vi "PicoScope6000ExampleStreaming.vi"() -> ()   [LabVIEW 2016]
uses:
  PS6000.dll
  Wrapper/ps6000Wrap/Release/ps6000Wrap.dll
panel:
  out "Triggered":bool
  in  "Acquisition Settings":T1={"Auto Stop"=TRUE, "Desired Sample Interval"=1, "Pre-trigger Samples"=0, "Post-trigger Samples"=1000000, "Down-Sample Ratio"=1, "Down-Sample Mode"=0, "Overview Buffer Size"=50000, "Time Units"=3} {"Time Units" items=["Nanoseconds (ns)"=2, "Microseconds (us)"=3, "Milliseconds (ms)"=4, "Seconds (s)"=5]; "Down-Sample Mode" items=["None"=0, "Aggregate"=1, "Average"=2, "Decimate"=4, "Distribution"=8]}
  in  "Channel A Settings":T2={"Enabled"=TRUE, "Coupling"=1, "Range"=7, "Analogue Offset"=0.0, "Bandwidth"=0} {"Bandwidth" items=["Full", "20 MHz"]; "Range" items=["10 mV", "20 mV", "50 mV", "100 mV", "200 mV", "500 mV", "1 V", "2 V", "5 V", "10 V", "20 V", "50 V ", "100 V"]; "Coupling" items=["AC", "DC 1 MOhm", "DC 50 Ohm"]}
  out "Sample Interval":u32
  out "Total Samples":u32
  in  "Trigger Settings":T3={"Trigger Enabled"=TRUE, "Trigger Source"=enum."Channel A", "Trigger Threshold (16-bit counts)"=0, "Trigger Direction"=2, "Trigger Delay (samples)"=0, "Auto Trigger Time (ms)"=5000} {"Trigger Direction" items=["Rising"=2, "Falling"=3]}
  out "Auto Stopped":bool
  in  "Apply Settings":bool
  out "Channel A":i16[](graph)
  in  "stop":bool
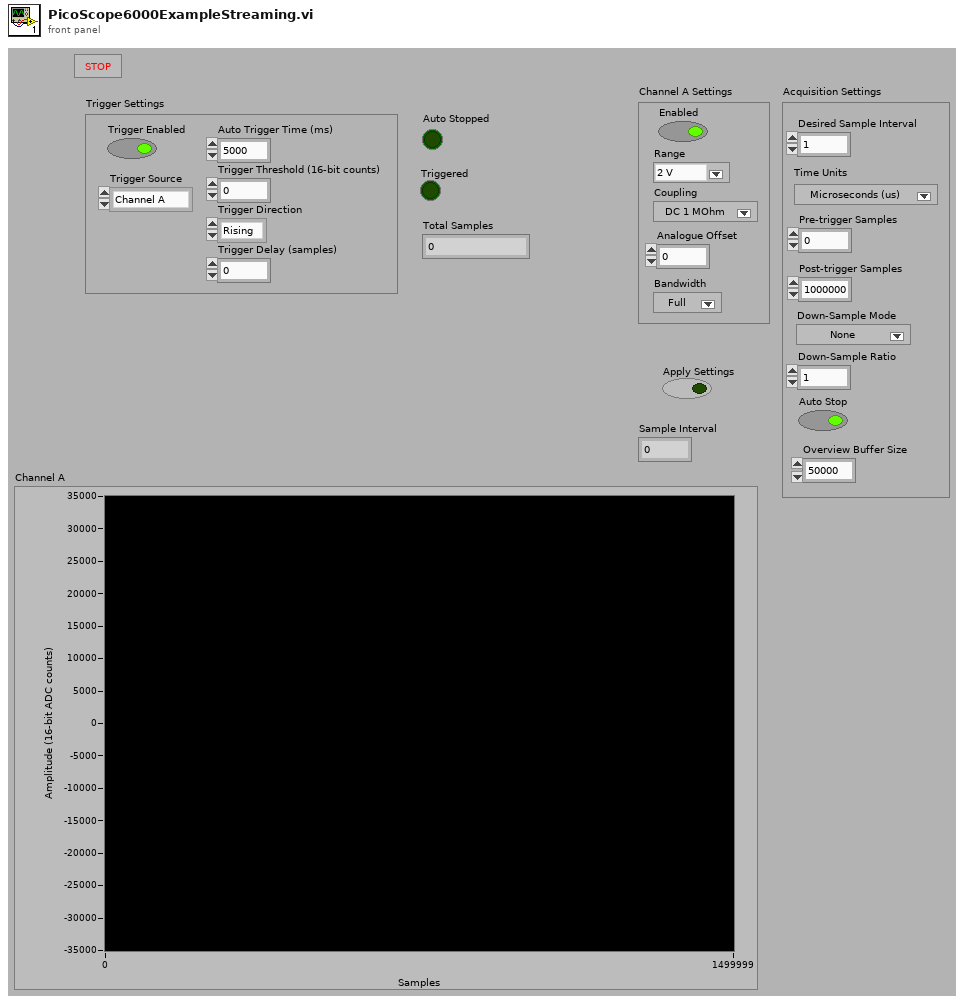
[diagram p1: front panel]
types:
  T1 = cluster{"Auto Stop":bool, "Desired Sample Interval":u32, "Pre-trigger Samples":u32, "Post-trigger Samples":u32, "Down-Sample Ratio":u32, "Down-Sample Mode":u32, "Overview Buffer Size":u32, "Time Units":u32}
  T2 = cluster{"Enabled":bool, "Coupling":u32, "Range":u32, "Analogue Offset":sgl, "Bandwidth":u32}
  T3 = cluster{"Trigger Enabled":bool, "Trigger Source":enum32{"Channel A", "Channel B", "Channel C", "Channel D"}, "Trigger Threshold (16-bit counts)":i16, "Trigger Direction":u16, "Trigger Delay (samples)":u32, "Auto Trigger Time (ms)":i16}
  T4 = cluster{"Enabled":bool, "Coupling":i32, "Range":u16, "Analogue Offset":sgl, "Bandwidth":i32}
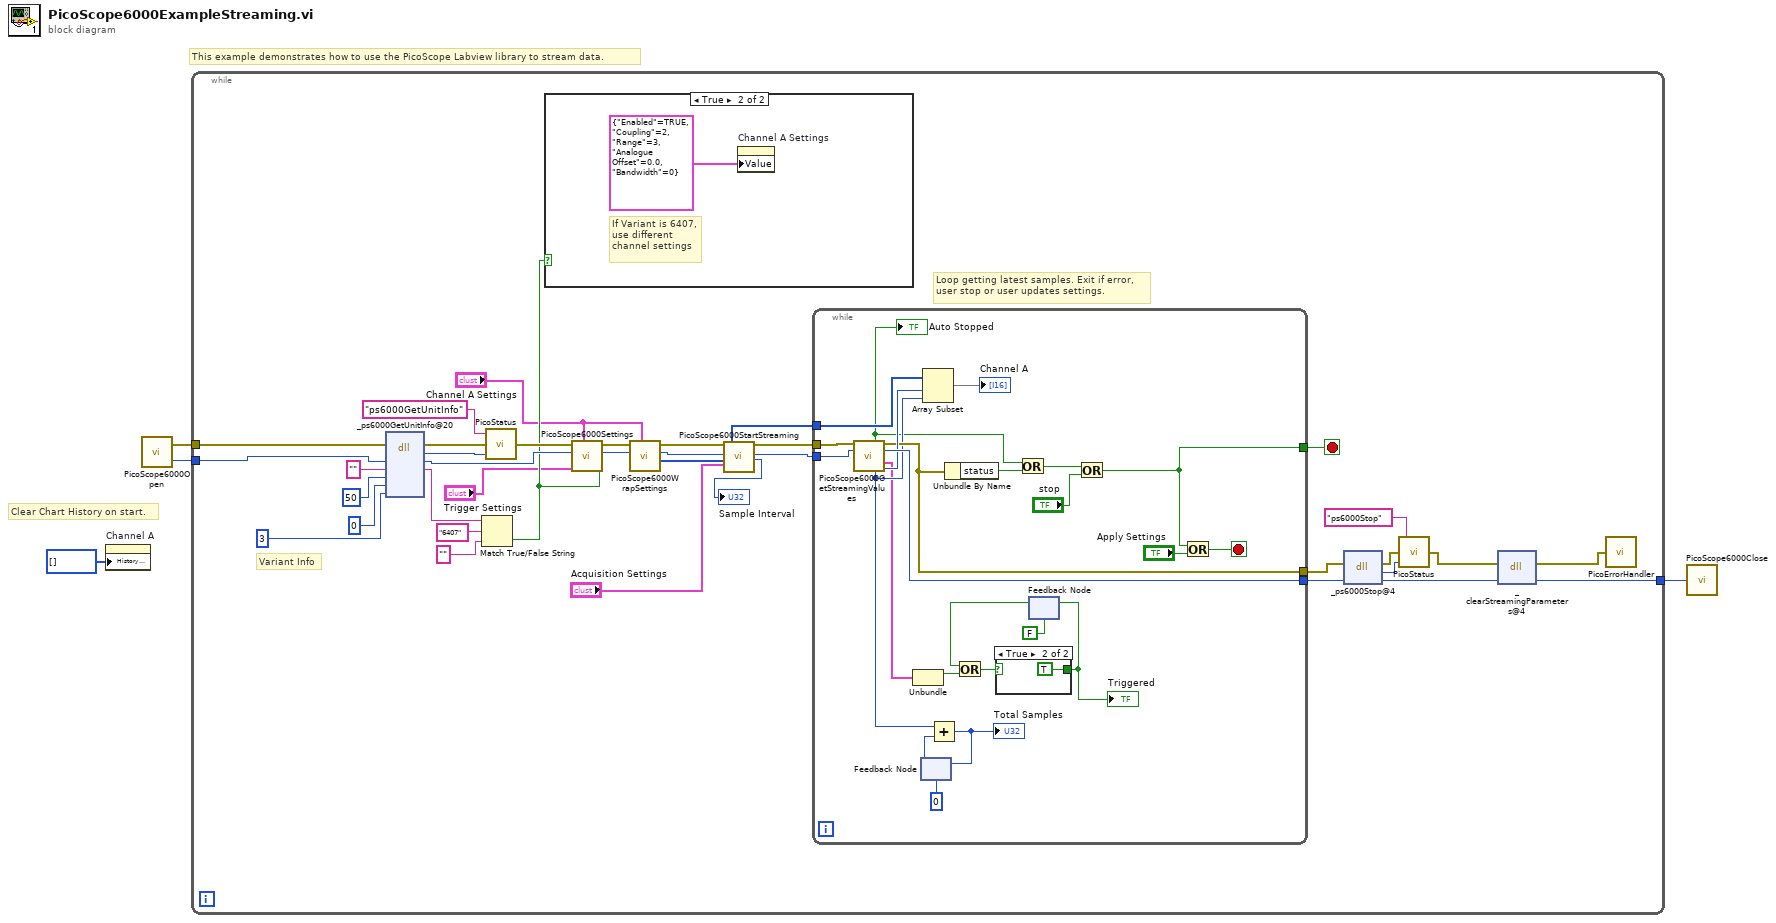
[diagram p0: block diagram]
diagram:
  # "Clear Chart History on start."
  # "This example demonstrates how to use the PicoScope Labview library to stream data."
  n1 = property on="Channel A" class="WFChart (strict)"("History Data"=i16[] []) -> ()  [unwired: 2 in, 2 out]
  n2 = call "PicoScope6000Open.vi"() -> ("error out"=w4:errorcluster, "handle"=w3:i16)  [unwired: 1 in]
  n3 = while {
    tunnel: [w8] -> w2
    tunnel: w4 -> [w27]
    tunnel: w3 -> [w26]
    stop <- w41 stop-if-true
    # "Variant Info"
    # "Loop getting latest samples. Exit if error, \nuser stop or user updates settings."
    n4 = dll-call lib="PS6000.dll" fn="_ps6000GetUnitInfo@20"(error in=w27, "handle"=w26, "string"="", "stringLength"=i16 50, "reqSize"=i16 0, "PICO_INFO"=u32 3 ("info")) -> (error out=w31:errorcluster, "PICO_STATUS"=w30:u32, "handle"=w25:i16, "string"=w28:string)  [unwired: 5 in, 1 out]
    n5 = Match True/False String(2:"" ("false string"), 3:"6407" ("true string"), 4:w28) -> (0:w23:bool)  [unwired: 1 out]
    n6 = call "PicoStatus.vi"("PICO STATUS"=w30, "error in"=w31, "source"="ps6000GetUnitInfo") -> ("error out"=w24:errorcluster)
    n7 = case shown="True" w23 {
      frame False {
      }
      frame True {
        # "If Variant is 6407,\nuse different \nchannel settings"
        n8 = property on="Channel A Settings" class="Clust (strict)"("Value"=T4 {"Enabled"=TRUE, "Coupling"=2, "Range"=3, "Analogue Offset"=0.0, "Bandwidth"=0} ("Channel A Settings")) -> ()  [unwired: 2 in, 2 out]
      }
    }
    n9 = call "PicoScope6000Settings.vi"("PS6407?"=w23, "Channel A Settings"="Channel A Settings", "Trigger Settings"="Trigger Settings", "handle in"=w25, "error in"=w24) -> ("handle out"=w15:i16, "error out"=w17:errorcluster)  [unwired: 5 in]
    n10 = call "PicoScope6000WrapSettings.vi"("Channel A Settings"="Channel A Settings", "Handle In"=w15, "error in (no error)"=w17) -> ("enabledChannels"=w5:i16[], "Handle Out"=w14:i16, "error out"=w16:errorcluster)  [unwired: 6 in]
    n11 = call "PicoScope6000StartStreaming.vi"("error in"=w16, "handle in"=w14, "Enabled Channels"=w5, "Acquisition Settings"="Acquisition Settings") -> ("Channel A"=w38:i16[], "error out"=w40:errorcluster, "handle out"=w39:i16, "Sample Interval"=→"Sample Interval":u32)  [unwired: 5 in, 7 out]
    n12 = while {
      tunnel: w40 -> [w60]
      tunnel: [w59] -> w22
      tunnel: [w64] -> w41
      tunnel: w38 -> [w62]
      tunnel: w39 -> [w61]
      tunnel: [w55] -> w21
      stop <- w63 stop-if-true
      n13 = call "PicoScope6000GetStreamingValues.vi"("error in"=w60, "handle in"=w61) -> ("Auto Stopped"=w50:bool, "error out"=w55:errorcluster, "handle out"=w59:i16, "Trigger"=w44:cluster{bool, "triggeredAt":u32}, "Number of Samples"=w52:u32, "Start Index"=w58:u32)  [unwired: 8 in]
      "Auto Stopped" <- w50
      n14 = Unbundle(w44) -> (w45:bool)  [unwired: 1 out]
      n15 = feedback #1(u32 0) -> (w53:u32)
      n16 = Array Subset(array=w62, index=w58, length=w52) -> (→"Channel A":i16[])
      n17 = Add(x=w52, y=w53) -> (x+y=w51:u32)
      "Total Samples" <- w51
      n18 = feedback-in #1(w51) -> ()
      n19 = Unbundle By Name(w55) -> ("status"=w56:bool)
      n20 = Or(x=w50, y=w56) -> (x .or. y?=w57:bool)
      n21 = feedback #2(FALSE) -> (w48:bool)
      n22 = Or(x=w48, y=w45) -> (x .or. y?=w47:bool)
      n23 = case shown="True" w47 {
        selector: w47 -> [w67 _]
        tunnel: [w67 TRUE] -> w49
        frame False {
        }
        frame True {
        }
      }
      "Triggered" <- w49
      n24 = feedback-in #2(w49) -> ()
      n25 = Or(x=w57, y="stop") -> (x .or. y?=w64:bool)
      n26 = Or(x=w64, y="Apply Settings") -> (x .or. y?=w63:bool)
    }
    n27 = dll-call lib="PS6000.dll" fn="_ps6000Stop@4"(error in=w21, "handle"=w22) -> (error out=w20:errorcluster, "PICO_STATUS"=w19:u32, "handle"=w9:i16)  [unwired: 2 in, 1 out]
    n28 = call "PicoStatus.vi"("PICO STATUS"=w19, "error in"=w20, "source"="ps6000Stop") -> ("error out"=w11:errorcluster)
    n29 = dll-call lib="D:/SoftwareFiles/LabVIEW Files/Picoscope/picoscope-master/sdk/6000/Wrapper/ps6000Wrap/Release/ps6000Wrap.dll" fn="_clearStreamingParameters@4" label="clearStreamingParameters"(error in=w11, "handle"=w9) -> (error out=w10:errorcluster, "handle"=w8:i16)  [unwired: 3 in, 1 out]
    n30 = call "PicoErrorHandler.vi"("error in"=w10) -> ()  [unwired: 1 out]
  }
  n31 = call "PicoScope6000Close.vi"("handle"=w2) -> ()
